vi "Unbundle.vi"() -> ()   [LabVIEW 2016]
panel:
  out "element":dbl
  out "String":string
  out "Boolean":bool
  out "Numeric":dbl
  in  "Cluster":T1
  in  "Array":dbl[](array[numeric])
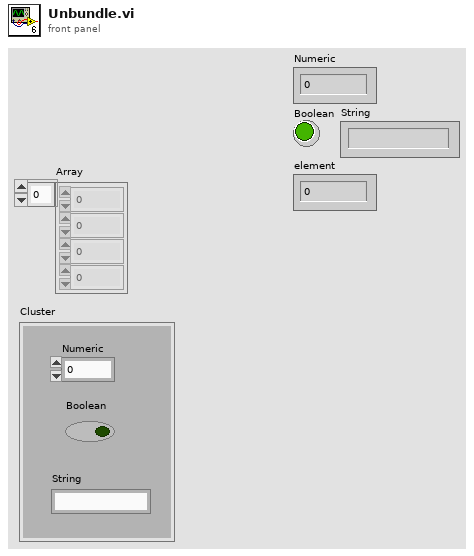
[diagram p1: front panel]
types:
  T1 = cluster{"Numeric":dbl, "Boolean":bool, "String":string}
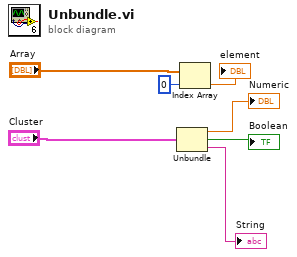
[diagram p0: block diagram]
diagram:
  n1 = Unbundle("Cluster") -> ("Numeric"=→"Numeric":dbl, "Boolean"=→"Boolean":bool, "String"=→"String":string)
  n2 = Index Array(array="Array", index=0) -> (element=→"element":dbl)
